vi "CM-Save Connector Type.vi"(0 "configuration file path":path=path "C:/PXI Connections.txt", 5 "Device":string="Use BNC-2090", 9 "ConType":T1, 11 "error in (no error)":errorcluster) -> (4 "file path":path, 15 "error out":errorcluster)   [LabVIEW 2020]
uses:
  Type Defs/PXISlot XControl/Connector Type.ctl
  <vilib>/Utility/config.llb/Write Key (String).vi
  <vilib>/Utility/config.llb/NI_LVConfig.lvlib
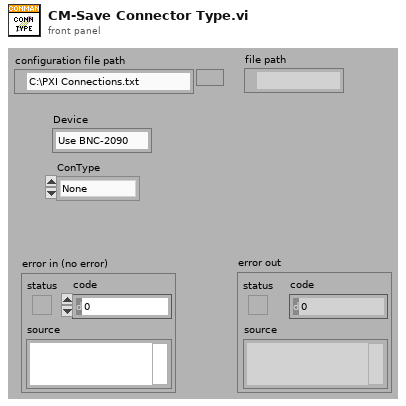
[diagram p1: front panel]
types:
  T1 = typedef "Connector Type.ctl" = enum16{"None", "PXI-4461", "BNC-2110", "BNC-2090", "PXIe-4463", "PXIe-4464"}
  T2 = typedef "NI_LVConfig.lvlib/Config Data RefNum.ctl" = refnum<k1>
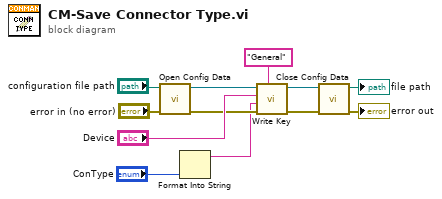
[diagram p0: block diagram]
diagram:
  n1 = call <vilib>:"Open Config Data.vi"("error in (no error)"="error in (no error)", "configuration file path"="configuration file path") -> ("error out"=w4:errorcluster, "refnum"=w5:T2)  [unwired: 7 in, 1 out]
  n2 = Format Into String("ConType") -> (resulting string=w1:string)  [unwired: 3 in, 1 out]
  n3 = call-poly <vilib>:"Write Key.vi"("section"="General", "error in (no error)"=w4, "value"=w1, "key"="Device", "refnum"=w5) -> ("error out"=w8:errorcluster, "refnum out"=w7:T2)  [unwired: 4 in, 1 out]
  n4 = call <vilib>:"Close Config Data.vi"("error in (no error)"=w8, "refnum"=w7) -> ("error out"=→"error out":errorcluster, "file path"=→"file path":path)  [unwired: 8 in]
